vi "Combine TDMS File To Another.vi"(8 "error in (no error)":errorcluster, 9 "Delete Index":bool, 10 "TDMS File 2":path, 11 "TDMS File 1":path) -> (0 "error out":errorcluster, 3 "Success?":bool)   [LabVIEW 2015]
doc: "This VI will append a TDMS file to an existing TDMS file and optionally delete the index from the combined file. This will take <B>TDMS File 2</b> and append it to the end of <b>TDMS File 1</b>. If the combine operation performed a successful copy then the <b>Success?</b> will be <b>TRUE</b>. Note that this simply means the merge was successful, it does not mean the output is valid.\n\n-----\nBrian Hoover (Hooovahh)"
uses:
  <vilib>/dlg_ctls.llb/Space Constant.vi
  <vilib>/Platform/system.llb/System Exec.vi
  <vilib>/Utility/error.llb/Trim Whitespace.vi
  <userlib>/_OpenG.lib/file/file.llb/Convert File Extension (Path)__ogtk.vi
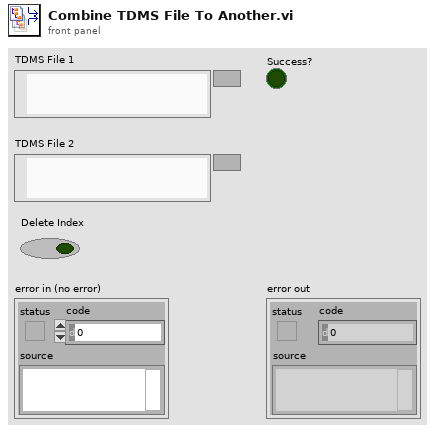
[diagram p1: front panel]
types:
  T1 = enum16{"open", "replace", "create", "open or create", "replace or create", "replace or create with confirmation"}
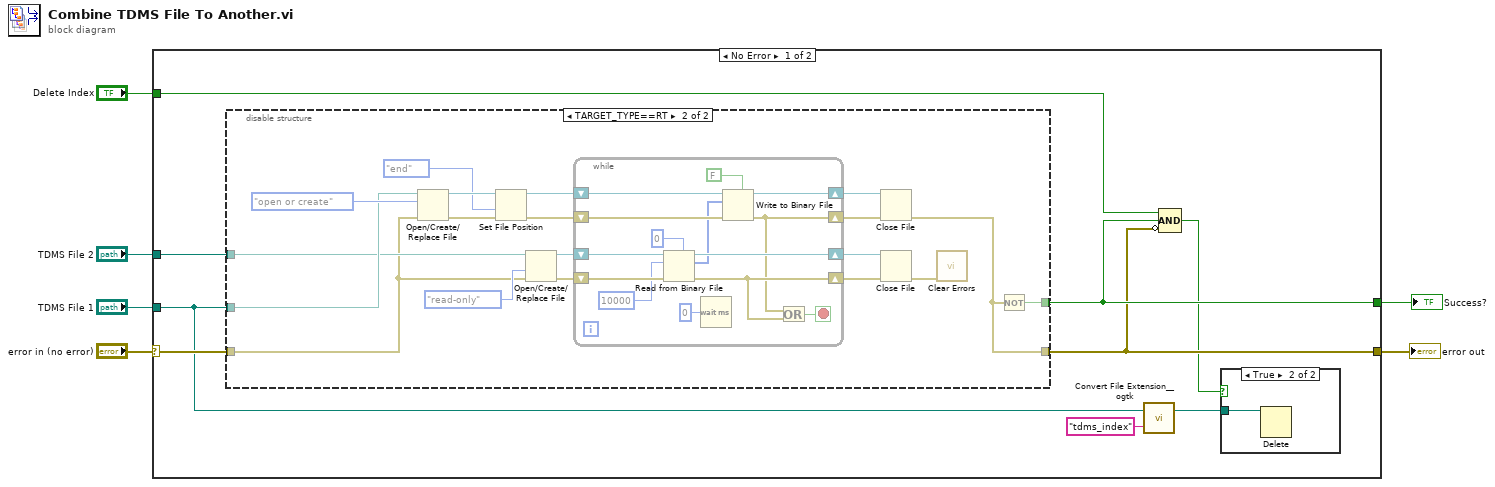
[diagram p0: block diagram]
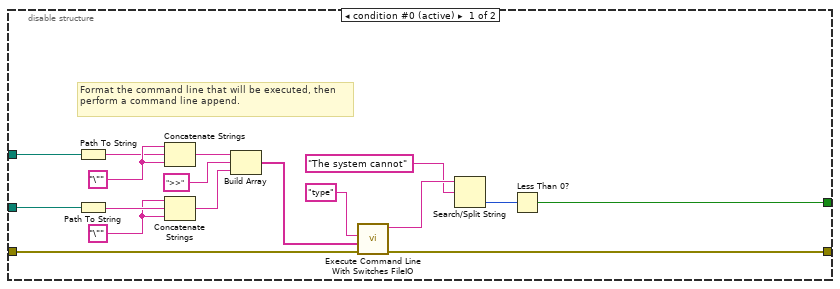
[diagram p3: hidden frame]
diagram:
  n1 = case shown="No Error" "error in (no error)" {
    selector: "error in (no error)" -> [w15 w67]
    tunnel: [w9 w67] -> w6
    tunnel: "TDMS File 2" -> [w14 _]
    tunnel: "TDMS File 1" -> [w7 _]
    tunnel: [w10 _] -> w3
    tunnel: "Delete Index" -> [w11 _]
    frame No Error {
      n2 = disable-structure shown="TARGET_TYPE==RT" {
        disable-tunnel: w15 -> [w32 w34]
        disable-tunnel: w14 -> [w20 w48]
        disable-tunnel: [w19 w40] -> w10
        disable-tunnel: [w18 w39] -> w9
        disable-tunnel: w7 -> [w17 w49]
        frame condition #0 (active) {
          w26 = "\"" ("string")
          w31 = "\"" ("string")
          # "Format the command line that will be executed, then perform a command line append."
          n3 = Path To String(path=w20) -> (string=w25:string)
          n4 = Path To String(path=w17) -> (string=w33:string)
          n5 = Concatenate Strings(w26, w25, w26) -> (w24:string)
          n6 = Concatenate Strings(w31, w33, w31) -> (w23:string)
          n7 = Build Array(w24, ">>" ("element"), w23) -> (w21:string[])
          n8 = call "Execute Command Line With Switches FileIO.vi"("error in (no error)"=w32, "Command Line Switches"=w21, "Command (dir)"="type") -> ("error out"=w18:errorcluster, "Standard Output"=w29:string)  [unwired: 7 in]
          n9 = Search/Split String(string=w29, search string/char (-)="The system cannot") -> (offset of match=w27:i32)  [unwired: 1 in, 2 out]
          n10 = Less Than 0?(x=w27) -> (x < 0?=w19:bool)
        }
        frame condition #1 {
          n11 = Open/Create/Replace File(file path (use dialog)=w49, error in=w34, operation (0:open)=T1."open or create") -> (refnum out=w37:refnum<file>, error out=w50:errorcluster)  [unwired: 3 in, 1 out]
          n12 = Set File Position(refnum=w37, from (0:start)=enum16{"start", "end", "current"}."end", error in=w50) -> (refnum out=w36:refnum<file>, error out=w38:errorcluster)  [unwired: 1 in]
          n13 = Open/Create/Replace File(file path (use dialog)=w48, error in=w34, access (0:read/write)=enum16{"read/write", "read-only", "write-only"}."read-only") -> (refnum out=w47:refnum<file>, error out=w46:errorcluster)  [unwired: 3 in, 1 out]
          n14 = while {
            shift-right: [w64] -> w45
            shift-left: w47 -> [w66]
            shift-right: [w58] -> w44
            shift-left: w46 -> [w65]
            shift-right: [w61] -> w51
            shift-left: w36 -> [w63]
            shift-right: [w56] -> w41
            shift-left: w38 -> [w62]
            stop <- w57 stop-if-true
            n15 = Read from Binary File(5:u8 0, 8:w65, 10:10000 ("count (1)"), 11:w66) -> (0:w58:errorcluster, 2:w60:u8[], 3:w64:refnum<file>)  [unwired: 2 in, 1 out]
            n16 = Wait (ms)(milliseconds to wait=u32 0) -> ()  [unwired: 1 out]
            n17 = Write to Binary File(file (use dialog)=w63, data=w60, error in=w62, 5:FALSE ("prepend array or string size? (T)")) -> (refnum out=w61:refnum<file>, error out=w56:errorcluster)  [unwired: 2 in, 1 out]
            n18 = Or(x=w56, y=w58) -> (x .or. y?=w57:bool)
          }
          n19 = Close File(refnum=w51, error in=w41) -> (error out=w39:errorcluster)  [unwired: 1 out]
          n20 = Close File(refnum=w45, error in=w44) -> (error out=w42:errorcluster)  [unwired: 1 out]
          n21 = call <vilib>:"Clear Errors.vi"("error in (no error)"=w42) -> ()  [unwired: 5 in, 2 out]
          n22 = Not(x=w39) -> (.not. x?=w40:bool)
        }
      }
      n23 = call-poly <userlib>:"Convert File Extension__ogtk.vi"("new ending (none)"="tdms_index", "file name"=w7) -> ("new filename"=w12:path)  [unwired: 1 out]
      n24 = Compound Arithmetic op=AND(w11, w10, invert w9) -> (w8:bool)
      n25 = case shown="True" w8 {
        tunnel: w12 -> [_ w16]
        frame False {
        }
        frame True {
          n26 = Delete(path (use dialog)=w16) -> ()  [unwired: 4 in, 3 out]
        }
      }
    }
    frame Error {
    }
  }
  "error out" <- w6
  "Success?" <- w3
